vi "Read Elevator Call.vi"(2 "Elevator Call":T1, 8 "error in (no error)":errorcluster, 11 "Interface Elevator in":refnum<class "Interface Elevator.lvclass">) -> (0 "error out":errorcluster, 3 "Interface Elevator out":refnum<class "Interface Elevator.lvclass">)   [LabVIEW 2022 SP3, in "Interface Elevator.lvclass"]
uses:
  Interface Elevator.lvclass
  Sim User Console Actor/Elevator Controller Actor/Elevator Call.ctl
  Sim User Console Actor/Elevator Controller Actor/Sim User Console Actor.lvclass
panel:
  # "Fourth Floor"
  # "Third Floor"
  # "Second Floor"
  # "First Floor"
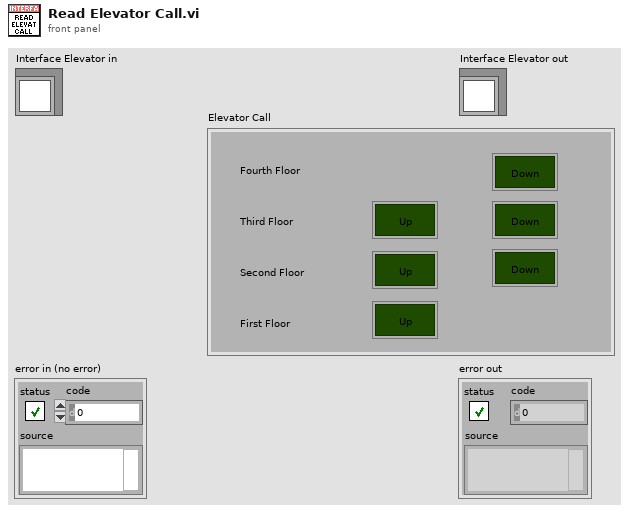
[diagram p1: front panel]
types:
  T1 = typedef "Sim User Console Actor.lvlib/Sim User Console Actor.lvclass/Elevator Call.ctl" = cluster{"Up":bool, "Up 2":bool, "Up 3":bool, "Down":bool, "Down 2":bool, "Down 3":bool}
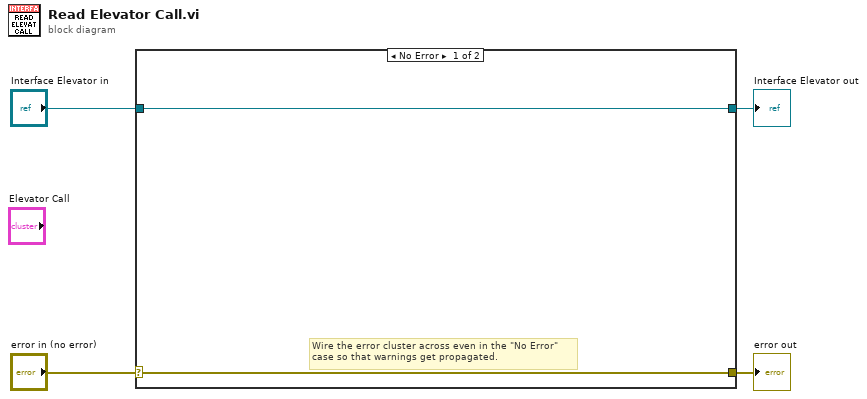
[diagram p0: block diagram]
diagram:
  n1 = case shown="No Error" "error in (no error)" {
    selector: "error in (no error)" -> [w5 w8]
    tunnel: [w5 w8] -> w3
    tunnel: [w6 w7] -> w1
    tunnel: "Interface Elevator in" -> [w6 w7]
    frame No Error {
      # "Wire the error cluster across even in the \"No Error\"\ncase so that warnings get propagated."
    }
    frame Error {
    }
  }
  "error out" <- w3
  "Interface Elevator out" <- w1
